vi "AlliGator Save FLI Dataset to HDF5 File v3 (VDM).vi"(5 "Compression (T)":bool=TRUE, 6 "Gate Names (Gate)":string[](array[string]), 7 "Software + Version":string, 8 "Error In":errorcluster, 9 "Dataset Information":T2={"Single Dataset Path"=path "", "Dataset ID in Series (1)"=1, "# Datasets in Series (1)"=1, "Dataset Timestamp (s)"=0.0, "Additional Metadata"="", "DAQ Parameters"={"# Pixel X"=0, "# Pixel Y"=0, "# Gates"=0, "# Datasets"=0, "Gate Image Exposure"=0.0, "Macrotime Gate Separation"=0.0, "Nanotime Gate Separation"=0.0, "Gate Width"=0.0, "Laser Period"=0.0, "SYNC Period"=0.0, "Gate Image Integration"=0.0}, "Dataset Data Description"="", "X Bin"=0, "Y Bin"=0}, 10 "Channel 2 Gate Image Array":T1[](array[typedef]), 11 "Channel 1 Gate Image Array":T1[](array[typedef])) -> (0 "Error Out":errorcluster, 3 "File Path out":path, 4 "Time (s)":dbl)   [LabVIEW 2021, in "AlliGator Files.lvlib"]
doc: "Save gate images (single- or dual-channel) and dataset information to HDF5 file."
uses:
  AlliGator Files.lvlib
  <vilib>/vision/Image Controls.llb/IMAQ Image.ctl
  AlliGator Saved Dataset Information.ctl
  Phasor/Phasor Fluorescence Lifetime Parameters v3.ctl
  <vilib>/addons/h5labview2/file/H5F.lvlib
  Time/Time.lvlib
  Error/Error.lvlib
  Phasor/Phasor.lvlib
panel:
  # "see the AlliGator License on the block diagram (Ctrl+E or Window:Show Block Diagram)"
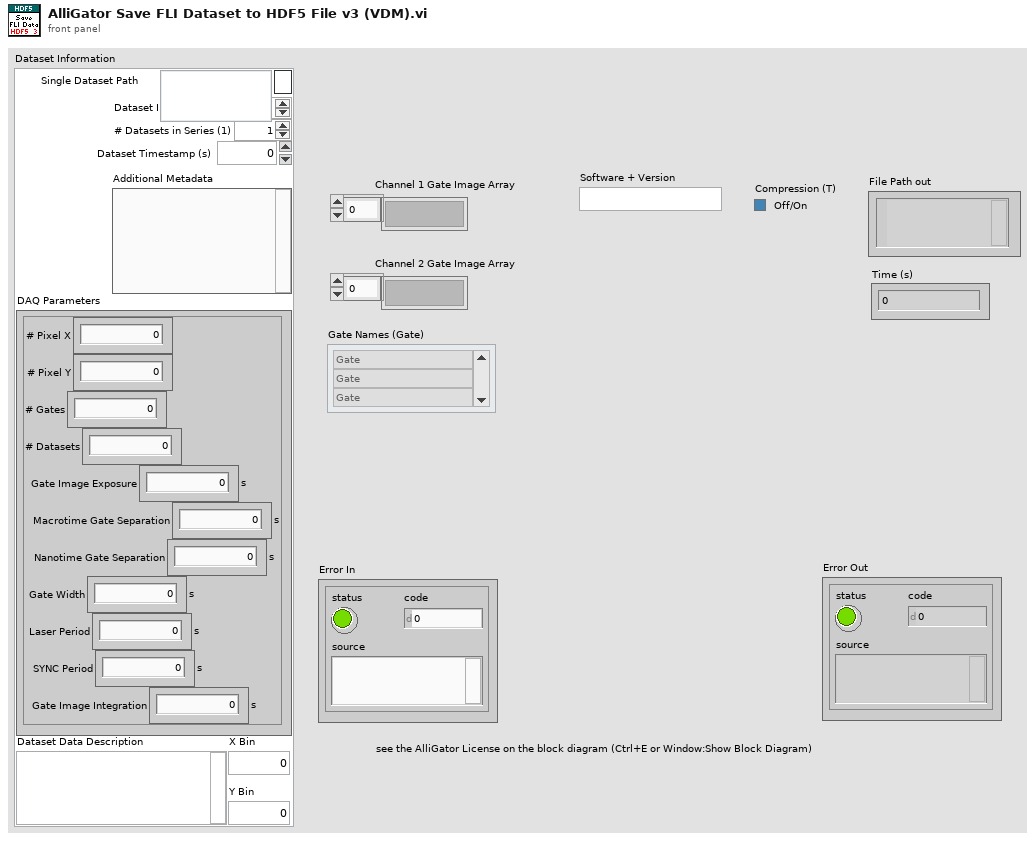
[diagram p1: front panel]
types:
  T1 = typedef "IMAQ Image.ctl" = refnum<image>
  T2 = typedef "AlliGator Files.lvlib/AlliGator Saved Dataset Information.ctl" = cluster{"Single Dataset Path":path, "Dataset ID in Series (1)":i32, "# Datasets in Series (1)":i32, "Dataset Timestamp (s)":dbl, "Additional Metadata":string, "DAQ Parameters":T3, "Dataset Data Description":string, "X Bin":i32, "Y Bin":i32}
  T3 = typedef "Phasor.lvlib/Phasor Fluorescence Lifetime Parameters v3.ctl" = cluster{"# Pixel X":i32, "# Pixel Y":i32, "# Gates":i32, "# Datasets":i32, "Gate Image Exposure":dbl[unit], "Macrotime Gate Separation":dbl[unit], "Nanotime Gate Separation":dbl[unit], "Gate Width":dbl[unit], "Laser Period":dbl[unit], "SYNC Period":dbl[unit], "Gate Image Integration":dbl[unit]}
  T4 = typedef "hid_t.ctl" = i64
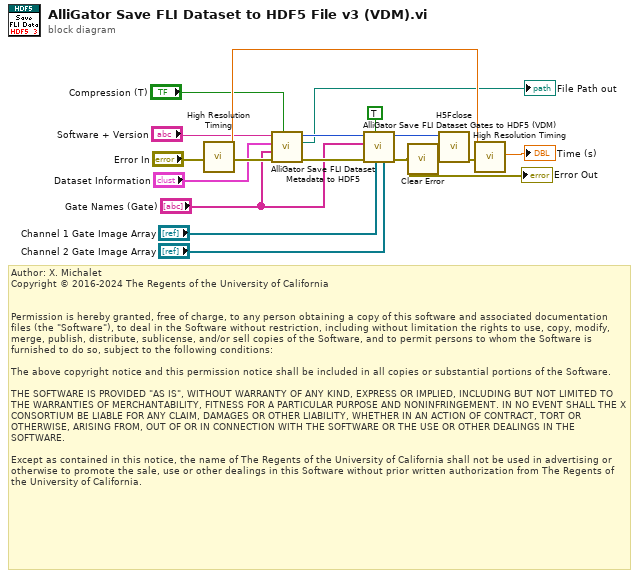
[diagram p0: block diagram]
diagram:
  # "Author: X. Michalet\nCopyright © 2016-2024 The Regents of the University of California\n \n\nPermission is hereby granted, free of charge, to any person obtaining a copy of this software and associated documentation files (the \"Software\"), to deal in the Software without restriction, including without limitation the rights to use, copy, modify, merge, publish, distribute, sublicense, and/or sell copies of the Software, and to permit persons to whom the Software is furnished to do so, subject to the following conditions:\n\nThe above copyright notice and this permission notice shall be included in all copies or substantial portions of the Software.\n\nTHE SOFTWARE IS PROVIDED \"AS IS\", WITHOUT WARRANTY OF ANY KIND, EXPRESS OR IMPLIED, INCLUDING BUT NOT LIMITED TO THE WARRANTIES OF MERCHANTABILITY, FITNESS FOR A PARTICULAR PURPOSE AND NONINFRINGEMENT. IN NO EVENT SHALL THE X CONSORTIUM BE LIABLE FOR ANY CLAIM, DAMAGES OR OTHER LIABILITY, WHETHER IN AN ACTION OF CONTRACT, TORT OR OTHERWISE, ARISING FROM, OUT OF OR IN CONNECTION WITH THE SOFTWARE OR THE USE OR OTHER DEALINGS IN THE SOFTWARE.\n\nExcept as contained in this notice, the name of The Regents of the University of California shall not be used in advertising or otherwise to promote the sale, use or other dealings in this Software without prior written authorization from The Regents of the University of California."
  n1 = call "High Resolution Timing.vi"("Error In"="Error In") -> ("elapsed (relative) seconds"=w15:dbl, "Error Out"=w16:errorcluster)  [unwired: 16 in, 1 out]
  n2 = call "AlliGator Save FLI Dataset Metadata to HDF5.vi"("Compression"="Compression (T)", "error in (no error)"=w16, "Gate Names"="Gate Names (Gate)", "Dataset Information"="Dataset Information", "Software + Version"="Software + Version") -> ("error out"=w7:errorcluster, "File Path out"=→"File Path out":path, "HDF5 File ref out"=w3:T4)  [unwired: 4 in]
  n3 = call "AlliGator Save FLI Dataset Gates to HDF5 (VDM).vi"("Channel 2 Gate Image Array"="Channel 2 Gate Image Array", "Channel 1 Gate Image Array"="Channel 1 Gate Image Array", "replace?"=TRUE, "error in (no error)"=w7, "Gate Names"="Gate Names (Gate)", "HDF5 File ref in"=w3) -> ("error out"=w12:errorcluster, "HDF5 File ref out"=w10:T4)  [unwired: 4 in]
  "Error Out" <- w12
  n4 = call "Clear Error.vi"("Error In"=w12) -> ("no Error Out"=w13:errorcluster)  [unwired: 8 in]
  n5 = call <vilib>:"H5Fclose.vi"("error in (no error)"=w13, "ref"=w10) -> ("error out"=w18:errorcluster)  [unwired: 9 in]
  n6 = call "High Resolution Timing.vi"("relative seconds (NaN)"=w15, "Error In"=w18) -> ("elapsed (relative) seconds"=→"Time (s)":dbl)  [unwired: 15 in, 2 out]
